vi "Actor Core.vi"(8 "error in (no error)":errorcluster, 11 "Common Measurements Interface in":refnum<class "Common Measurements Interface.lvclass">) -> (0 "error out":errorcluster, 3 "Actor Framework.lvlib:Actor":refnum<class "Actor.lvclass">)   [LabVIEW 2015, in "Common Measurements Interface.lvclass"]
uses:
  Common Measurements Interface.lvclass
  <vilib>/ActorFramework/Actor/Actor.lvclass
  Queued Listbox/Queued Listbox.xctl
  Common Measurements Interface.lvclass/Common Measurements Interface.ctl
  Mag Lab Measure Interface/Mag Lab Measure UI.lvclass/Mag Lab Measure UI.ctl
  <vilib>/ActorFramework/Actor/Actor.lvclass/Actor.ctl
  <vilib>/ActorFramework/Message Enqueuer/Message Enqueuer.lvclass/Message Enqueuer.ctl
  Mag Lab Graph/MagLabGraph.lvclass
  Mag Lab Measure Base Messages/Launch graph Msg/Launch graph Msg.lvclass/Launch graph Msg.ctl
  Mag Lab Measure Controller Messages/Start measurements Msg/Start measurements Msg.lvclass/Start measurements Msg.ctl
  Mag Lab Measure Controller Messages/Pause measurements Msg/Pause measurements Msg.lvclass/Pause measurements Msg.ctl
  <vilib>/ActorFramework/Message Enqueuer/Init from Existing Queue.vi
  <vilib>/ActorFramework/Message Enqueuer/Enqueue.vi
  <vilib>/ActorFramework/Message Priority Queue/Priority Enqueue.vi
  <vilib>/ActorFramework/Message Enqueuer/Message Enqueuer.lvclass
  <vilib>/ActorFramework/Stop Msg/Stop Msg.lvclass
  Mag Lab Measure Base Messages/Launch graph Msg/Launch graph Msg.lvclass
  Mag Lab Measure Controller Messages/Start measurements Msg/Start measurements Msg.lvclass
  Mag Lab Measure Controller Messages/Pause measurements Msg/Pause measurements Msg.lvclass
  Mag Lab Measure Controller Messages/Stop all measurements Msg/Stop all measurements Msg.lvclass
  Mag Lab Measure Interface/Interface with menu/Interface with menu.lvclass
  Mag Lab Measure Interface/Mag Lab Measure UI.lvclass
  Mag Lab Error Handler/Mag Lab Error Handler.lvclass
panel:
  in  "Syncronize measurements":bool=TRUE
  in  "Pause":bool
  in  "Repeat times":i32=-1
  in  "Time Stamp":timestamp
  in  "Stop":bool
  out "File Path":path
  in  "Graph":bool
  in  "Run":bool
  in  "Measure":string[](xcontrol)
  out "Name":string
  in  "Parameters":cluster{"Text":string}
  out "Log":string
  in  "Exit":bool
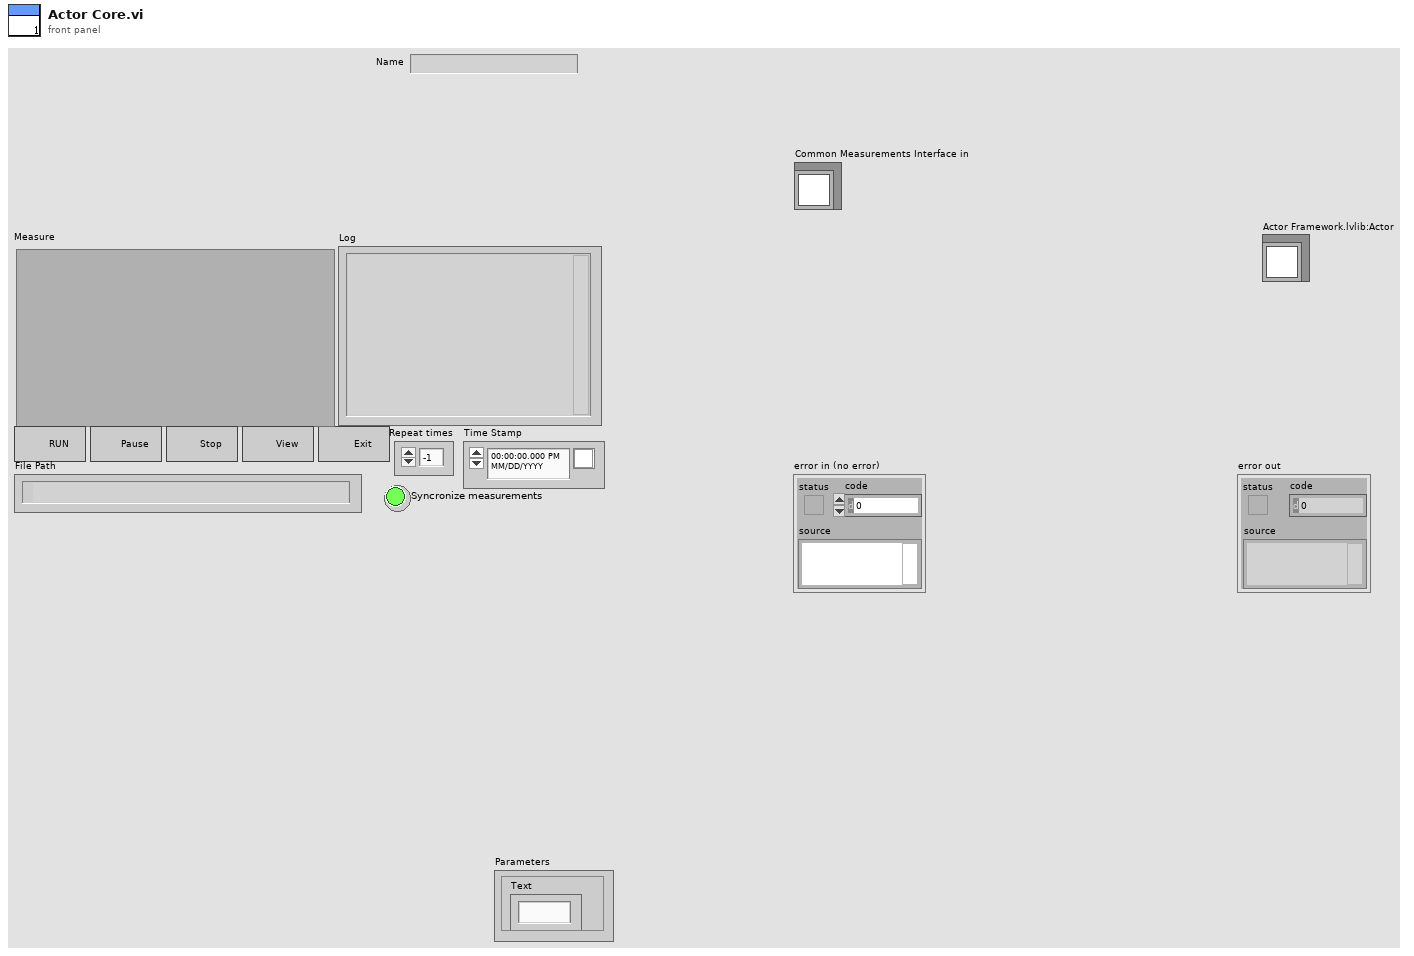
[diagram p1: front panel]
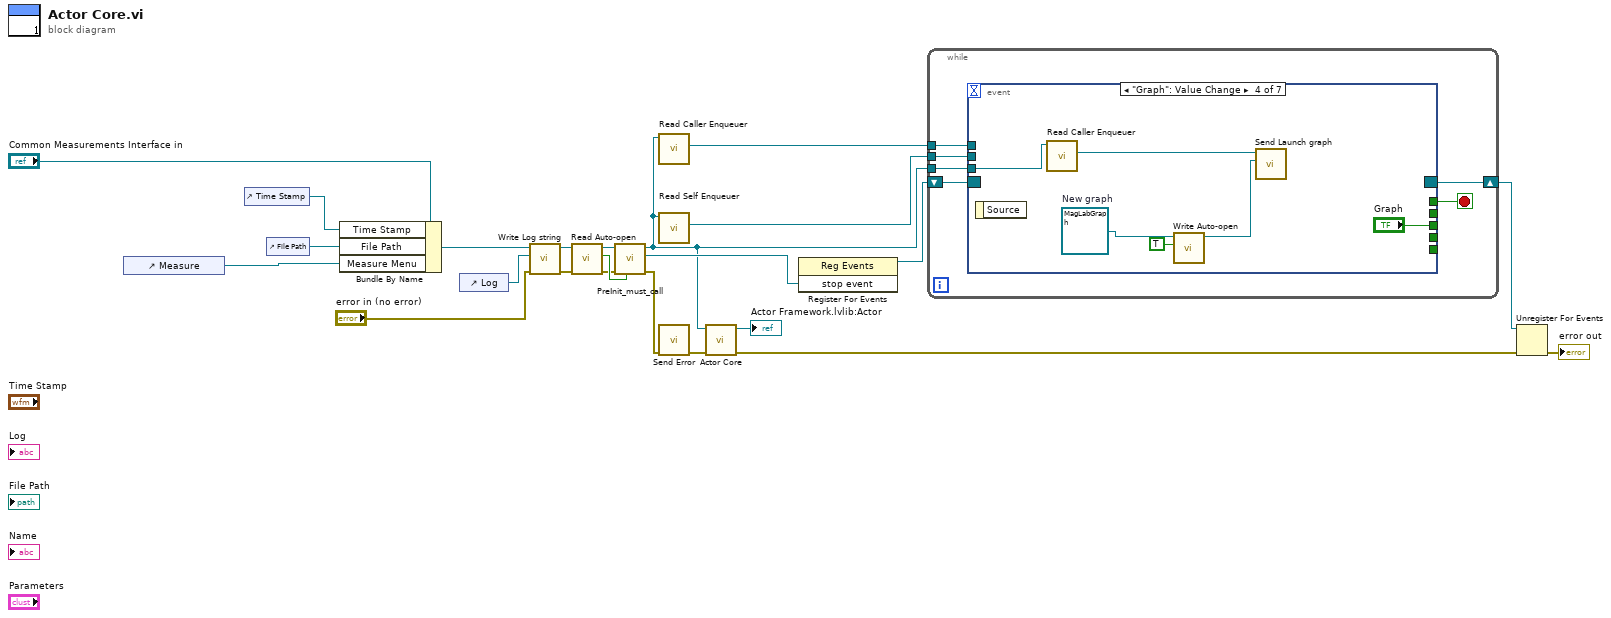
[diagram p0: block diagram]
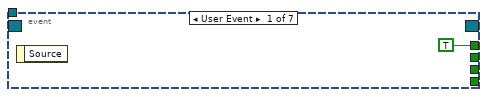
[diagram p2: hidden frame]
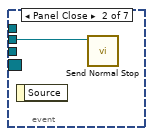
[diagram p3: hidden frame]
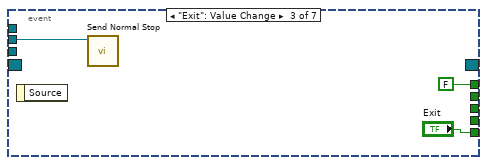
[diagram p4: hidden frame]
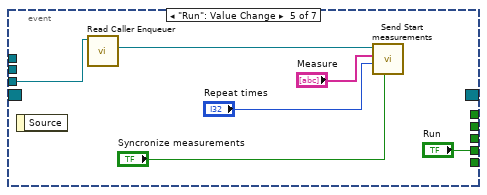
[diagram p5: hidden frame]
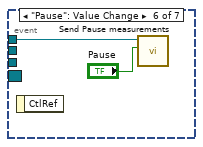
[diagram p6: hidden frame]
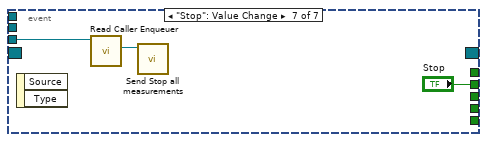
[diagram p7: hidden frame]
diagram:
  n1 = control-ref of="Measure"() -> (w14:refnum<vi>)
  n2 = control-ref of="Time Stamp"() -> (w8:refnum<vi>)
  n3 = control-ref of="File Path"() -> (w9:refnum<vi>)
  n4 = Bundle By Name(cluster="Common Measurements Interface in", "Time Stamp"=w8, "File Path"=w9, "Measure Menu"=w14) -> (w15:refnum<class "Common Measurements Interface.lvclass">)
  n5 = control-ref of="Log"() -> (w20:refnum<vi>)
  n6 = call "Write Log string.vi"("error in (no error)"="error in (no error)", "Log string"=w20, "Mag Lab Measure Interface in"=w15) -> ("error out"=w4:errorcluster, "Mag Lab Measure Interface out"=w7:refnum<class "Common Measurements Interface.lvclass">)  [unwired: 7 in]
  n7 = call "Read Auto-open.vi"("error in (no error)"=w4, "Mag Lab Measure UI in"=w7) -> ("error out"=w3:errorcluster, "Auto-open"=w5:bool, "Mag Lab Measure UI out"=w6:refnum<class "Common Measurements Interface.lvclass">)  [unwired: 7 in]
  n8 = call-dynamic "PreInit_must_call.vi"("Open Actor Core front panel? (T)"=w5, "error in (no error)"=w3, "Mag Lab Measure Interface in"=w6) -> ("error out"=w13:errorcluster, "stop event"=w21:refnum<user-event>, "Mag Lab Measure Interface out"=w2:refnum<class "Common Measurements Interface.lvclass">)  [unwired: 6 in]
  n9 = call <vilib>:"Read Caller Enqueuer.vi"("Actor"=w2) -> ("Caller Enqueuer"=w1:refnum<class "Message Enqueuer.lvclass">)  [unwired: 10 in]
  n10 = call <vilib>:"Read Self Enqueuer.vi"("Actor"=w2) -> ("Self Enqueuer"=w19:refnum<class "Message Enqueuer.lvclass">)  [unwired: 10 in]
  n11 = call "Send Error.vi"("error in (no error)"=w13) -> ("error out"=w18:errorcluster)  [unwired: 9 in, 1 out]
  n12 = call-parent "Actor Core.vi"("error in (no error)"=w18, "Mag Lab Measure Interface in"=w2) -> ("error out"=w10:errorcluster, "Actor Framework.lvlib:Actor"=→"Actor Framework.lvlib:Actor":refnum<class "Actor.lvclass">)  [unwired: 8 in]
  n13 = register-events(w21) -> (reference out=w22:refnum<event-registration>)  [unwired: 2 in, 1 out]
  n14 = while {
    tunnel: w19 -> [w27]
    shift-right: [w26] -> w11
    shift-left: w22 -> [w28]
    tunnel: w2 -> [w25]
    tunnel: w1 -> [w24]
    stop <- w29 stop-if-true
    n15 = event shown="[3] \"Graph\": Value Change" {
      selector: w28 -> [_ _ _ _ _ _ _]
      dyn-events: [_ _ _ _ _ _ _] -> w26
      timeout: _ -> [_ _ _ _ _ _ _]
      tunnel: [TRUE _ FALSE _ _ _ _] -> w29
      tunnel: w27 -> [_ w31 w32 _ _ _ _]
      tunnel: [_ _ "Exit" _ _ _ _] -> _
      tunnel: [_ _ _ _ "Run" _ _] -> _
      tunnel: w25 -> [_ _ _ w40 w45 _ w50]
      tunnel: [_ _ _ "Graph" _ _ _] -> _
      tunnel: [_ _ _ _ _ _ "Stop"] -> _
      tunnel: w24 -> [_ _ _ _ _ w47 _]
      event User Event {
        n16 = event-data() -> ()  [unwired: 1 in, 1 out]
      }
      event Panel Close {
        n17 = event-data() -> ()  [unwired: 1 in, 1 out]
        n18 = call <vilib>:"Send Normal Stop.vi"("Message Enqueuer"=w31) -> ()  [unwired: 10 in, 1 out]
      }
      event "Exit": Value Change {
        n19 = event-data() -> ()  [unwired: 1 in, 1 out]
        n20 = call <vilib>:"Send Normal Stop.vi"("Message Enqueuer"=w32) -> ()  [unwired: 10 in, 1 out]
      }
      event "Graph": Value Change {
        w37 = refnum<class "MagLabGraph.lvclass"> refnum  # New graph
        n21 = event-data() -> ()  [unwired: 1 in, 1 out]
        n22 = call <vilib>:"Read Caller Enqueuer.vi"("Actor"=w40) -> ("Caller Enqueuer"=w39:refnum<class "Message Enqueuer.lvclass">)  [unwired: 10 in]
        n23 = call "Write Auto-open.vi"("Auto-open"=TRUE, "Mag Lab Measure UI in"=w37) -> ("Mag Lab Measure UI out"=w36:refnum<class "MagLabGraph.lvclass">)  [unwired: 8 in, 1 out]
        n24 = call "Send Launch graph.vi"("MagLabGraph.lvclass"=w36, "Message Enqueuer"=w39) -> ()  [unwired: 8 in, 2 out]
      }
      event "Run": Value Change {
        n25 = event-data() -> ()  [unwired: 1 in, 1 out]
        n26 = call <vilib>:"Read Caller Enqueuer.vi"("Actor"=w45) -> ("Caller Enqueuer"=w44:refnum<class "Message Enqueuer.lvclass">)  [unwired: 10 in]
        n27 = call "Send Start measurements.vi"("Syncronize measurements"="Syncronize measurements", "Repeat times"="Repeat times", "Measurements"="Measure", "Message Enqueuer"=w44) -> ()  [unwired: 6 in, 2 out]
      }
      event "Pause": Value Change {
        n28 = event-data() -> ()  [unwired: 1 in, 1 out]
        n29 = call "Send Pause measurements.vi"("Pause"="Pause", "Message Enqueuer"=w47) -> ()  [unwired: 8 in, 2 out]
      }
      event "Stop": Value Change {
        n30 = event-data() -> ()  [unwired: 1 in, 2 out]
        n31 = call <vilib>:"Read Caller Enqueuer.vi"("Actor"=w50) -> ("Caller Enqueuer"=w49:refnum<class "Message Enqueuer.lvclass">)  [unwired: 10 in]
        n32 = call "Send Stop all measurements.vi"("Message Enqueuer"=w49) -> ()  [unwired: 9 in, 2 out]
      }
    }
  }
  n33 = Unregister For Events(event registration refnum=w11, error in=w10) -> (error out=→"error out":errorcluster)
